vi "EtherCAT Fault Updated.vi"(8 "error in":errorcluster, 10 "Fault Status":bool) -> (0 "error out":errorcluster)   [LabVIEW 2024, in "EtherCAT Model.lvlib"]
doc: "This updates the fault status\n_____\nCreated using DQMH Event Scripter 7.0.1.1316."
uses:
  EtherCAT Model.lvlib
  EtherCAT Fault Updated Argument--cluster.ctl
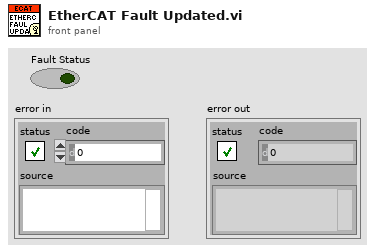
[diagram p1: front panel]
types:
  T1 = typedef "EtherCAT Model.lvlib/EtherCAT Fault Updated Argument--cluster.ctl" = cluster{"Boolean":bool, "Fault Status":bool}
  T2 = typedef "EtherCAT Model.lvlib/Broadcast Events--cluster.ctl" = cluster{"Module Did Init":refnum<user-event>, "Status Updated":refnum<user-event>, "Error Reported":refnum<user-event>, "Module Did Stop":refnum<user-event>, "Update Module Execution Status":refnum<user-event>, "Raw Data Updated":refnum<user-event>, "Date Updated":refnum<user-event>, "EtherCAT Connection Updated":refnum<user-event>, "EtherCAT Fault Updated":refnum<user-event>}
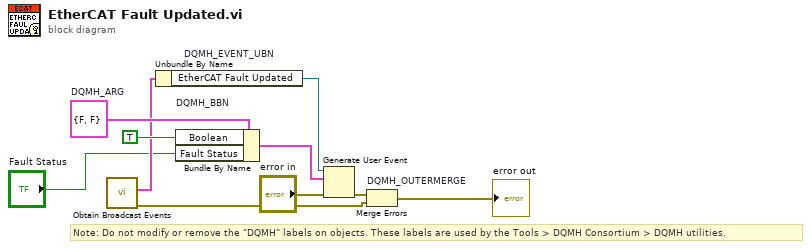
[diagram p0: block diagram]
diagram:
  w5 = T1 {"Boolean"=FALSE, "Fault Status"=FALSE}  # DQMH_ARG
  # "Note: Do not modify or remove the \"DQMH\" labels on objects. These labels are used by the Tools > DQMH Consortium > DQMH utilities."
  n1 = call "Obtain Broadcast Events.vi"() -> ("error out"=w3:errorcluster, "EtherCAT Model Broadcast Events"=w2:T2)  [unwired: 10 in]
  n2 = Unbundle By Name "DQMH_EVENT_UBN"(w2) -> ("EtherCAT Fault Updated"=w7:refnum<user-event>)
  n3 = Bundle By Name "DQMH_BBN"(cluster=w5, "Boolean"=TRUE, "Fault Status"="Fault Status") -> (w8:T1)
  n4 = Generate User Event(user event=w7, event data cluster=w8, error in="error in") -> (error out=w6:errorcluster)  [unwired: 1 in, 1 out]
  n5 = Merge Errors "DQMH_OUTERMERGE"(w6, w3) -> (→"error out":errorcluster)
